vi "Handshake.vi"(8 "error in":errorcluster, 10 "timeout ms (25000)":i32, 11 "RawSocket Handler in":refnum<class "RawSocket TCP Handler.lvclass">) -> (0 "error out":errorcluster, 3 "RawSocket Handler out":refnum<class "RawSocket TCP Handler.lvclass">)   [LabVIEW 2020, in "wamplv.lvlib" / "RawSocket TCP Handler.lvclass"]
uses:
  RawSocket TCP Handler.lvclass
  TypeDefs/Serilisation Types.ctl
  RawSocket TCP Handler.lvclass/RawSocket TCP Handler.ctl
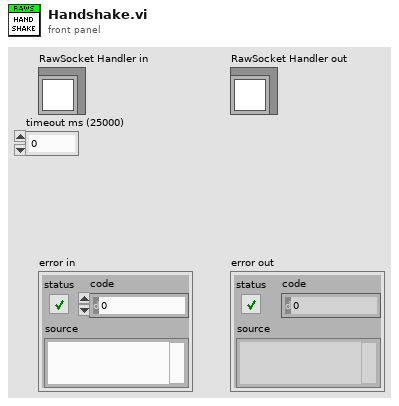
[diagram p1: front panel]
types:
  T1 = typedef "wamplv.lvlib/RawSocket TCP Handler.lvclass/Serilisation Types.ctl" = u8
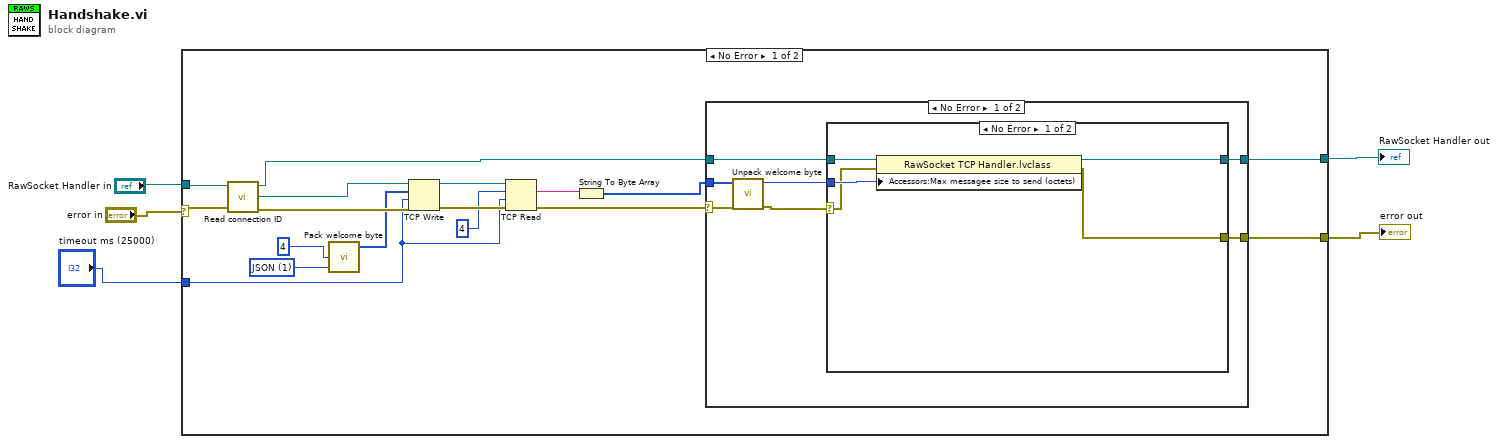
[diagram p0: block diagram]
diagram:
  n1 = case shown="No Error" "error in" {
    selector: "error in" -> [w21 w40]
    tunnel: [w7 w40] -> w4
    tunnel: [w8 w39] -> w5
    tunnel: "RawSocket Handler in" -> [w22 w39]
    tunnel: "timeout ms (25000)" -> [w6 _]
    frame No Error {
      w17 = T1 1 items=["JSON"=1, "MessagePack"=2] ("Serliaser")
      n2 = call-dynamic "Read connection ID.vi"("error in (no error)"=w21, "TCPSocketBasedCommHandlerBase in"=w22) -> ("error out"=w19:errorcluster, "connection ID"=w20:refnum<k5>, "TCPSocketBasedCommHandlerBase out"=w15:refnum<class "RawSocket TCP Handler.lvclass">)  [unwired: 7 in]
      n3 = call "Pack welcome byte.vi"("Serliaser"=w17, "Length (octets)"=u8 4) -> ("Bytes"=w16:u8[])  [unwired: 3 in]
      n4 = TCP Write(connection ID=w20, data in=w16, error in (no error)=w19, 9:w6) -> (connection ID out=w14:refnum<k5>, error out=w13:errorcluster)  [unwired: 1 out]
      n5 = TCP Read(connection ID=w14, bytes to read=4, error in (no error)=w13, 9:w6) -> (data out=w12:string, error out=w10:errorcluster)  [unwired: 1 in, 1 out]
      n6 = String To Byte Array(string=w12) -> (unsigned byte array=w11:u8[])
      n7 = case shown="No Error" w10 {
        selector: w10 -> [w29 w38]
        tunnel: w11 -> [w27 _]
        tunnel: w15 -> [w25 w37]
        tunnel: [w24 w37] -> w8
        tunnel: [w23 w38] -> w7
        frame No Error {
          n8 = call "Unpack welcome byte.vi"("error in"=w29, "Byte"=w27) -> ("error (out)"=w28:errorcluster, "Length (octets)"=w26:u8)  [unwired: 7 in, 1 out]
          n9 = case shown="No Error" w28 {
            selector: w28 -> [w31 w36]
            tunnel: w26 -> [w34 _]
            tunnel: w25 -> [w33 w35]
            tunnel: [w32 w35] -> w24
            tunnel: [w30 w36] -> w23
            frame No Error {
              n10 = property class="RawSocket TCP Handler.lvclass"(reference=w33, error in=w31, "Accessors:Max messagee size to send (octets)"=w34) -> (reference out=w32:refnum<class "RawSocket TCP Handler.lvclass">, error out=w30:errorcluster)
            }
            frame Error {
            }
          }
        }
        frame Error {
        }
      }
    }
    frame Error {
    }
  }
  "RawSocket Handler out" <- w5
  "error out" <- w4
